vi "get_qer.vi"(8 "error in (no error)":errorcluster, 11 "VISA Refnum in":refnum<visa-resource-name>) -> (0 "error out":errorcluster, 2 "QER":string, 3 "VISA Refnum out":refnum<visa-resource-name>)   [LabVIEW 2018]
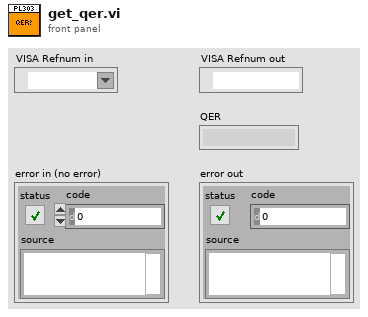
[diagram p1: front panel]
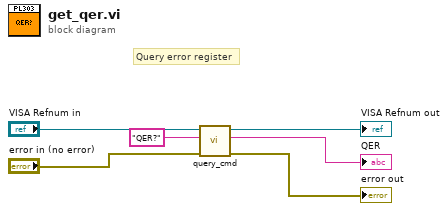
[diagram p0: block diagram]
diagram:
  # "Query error register"
  n1 = call "query_cmd.vi"("error in (no error)"="error in (no error)", "write buffer"="QER?", "VISA Refnum in"="VISA Refnum in") -> ("error out"=→"error out":errorcluster, "String"=→"QER":string, "VISA Refnum out"=→"VISA Refnum out":refnum<visa-resource-name>)  [unwired: 6 in]
